vi "Mock Stop Helper Loop from Process Loop.vi"(8 "error in (no error)":errorcluster, 9 "timeout in ms (-1)":i32, 11 "Mock Process in":refnum<class "Mock Process.lvclass">) -> (0 "error out":errorcluster, 1 "timed out?":bool, 3 "Mock Process out":refnum<class "Mock Process.lvclass">)   [LabVIEW 2020, in "Mock Process.lvclass"]
uses:
  Mock Process.lvclass
  Framework/Helper Loop/Helper Loop.lvclass
  Framework/Process/Process.lvclass
  C:/Users/anton/Documents/GitHub/Triarc-Framework/source/Framework/Process/Process.lvclass
  C:/Users/anton/Documents/GitHub/Triarc-Framework/source/Framework/Base/Base.lvclass
  C:/Users/anton/Documents/GitHub/Triarc-Framework/source/Framework/Error Handler Interface/Error Handler Interface.lvclass
  C:/Users/anton/Documents/GitHub/Triarc-Framework/source/Framework/Logging/Logging.lvclass
  C:/Users/anton/Documents/GitHub/Triarc-Framework/source/Framework Test/Mock Process/Mock Process.lvclass
  C:/Users/anton/Documents/GitHub/Triarc-Framework/source/Framework/Helper Loop/Helper Loop.lvclass
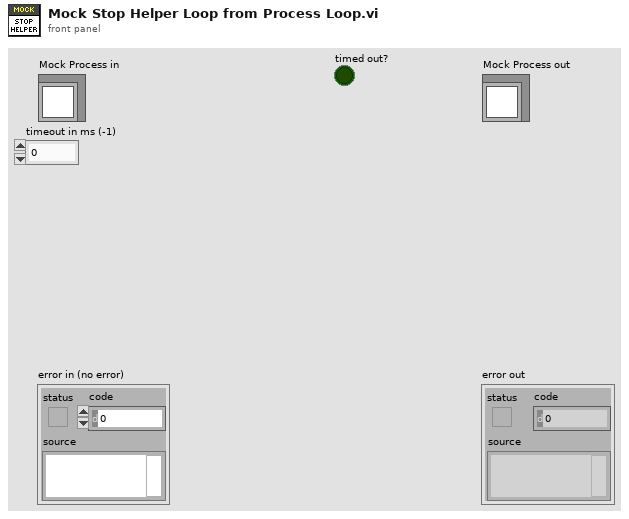
[diagram p1: front panel]
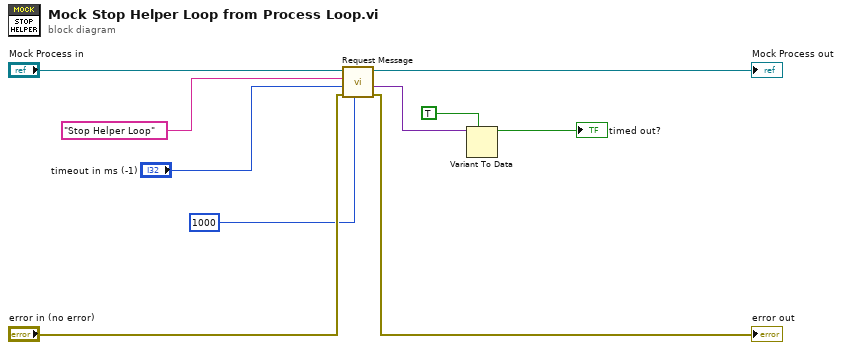
[diagram p0: block diagram]
diagram:
  n1 = call "Request Message.vi"("timeout in ms (-1)"=1000, "error in (no error)"="error in (no error)", "Request Message Data"="timeout in ms (-1)", "Request Message"="Stop Helper Loop", "Process In"="Mock Process in") -> ("error out"=→"error out":errorcluster, "Response Message Data"=w5:variant, "Process Out"=→"Mock Process out":refnum<class "Mock Process.lvclass">)  [unwired: 2 in, 2 out]
  n2 = Variant To Data(type=TRUE, Variant=w5) -> (data=→"timed out?":bool)  [unwired: 1 in, 1 out]
